vi "Navigation.vi"(0 "output angle":dbl, 4 "output xy":dbl, 6 "Debug":bool, 8 "GoTo Navigation":bool, 11 "IA State Output in":T1) -> (3 "IA State Output out":T1)   [LabVIEW 2018]
uses:
  Core/AI Input.ctl
  Core/AI Robot.ctl
  Intel/Functions Enum.ctl
  Intel/AttackerStates.ctl
  Path Planning/RRT/PathDests.ctl
  Path Planning/RRT/PathDest.ctl
  Core/AI Ball.ctl
  Core/Field Size.ctl
  Core/AI Judge.ctl
  Intel/Command Enum.ctl
  Util/Events/Events.ctl
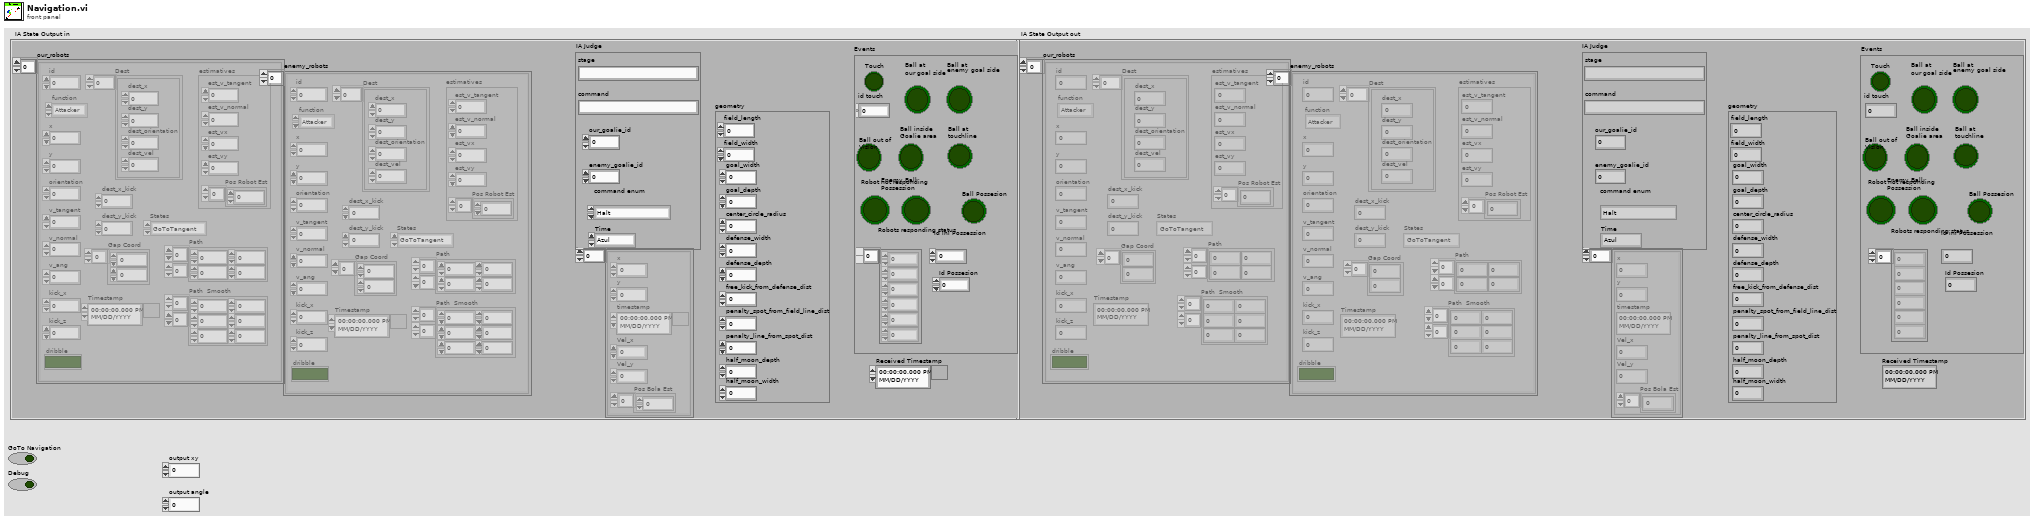
[diagram p1: front panel]
types:
  T1 = typedef "AI Input.ctl" = cluster{"our_robots":T2[], "enemy_robots":T2[], "balls":T7[], "geometry":T8, "IA Judge":T9, "Received Timestamp":timestamp, "Events":T11}
  T2 = typedef "AI Robot.ctl" = cluster{"id":u32, "function":T3, "x":dbl, "y":dbl, "orientation":dbl, "v_tangent":dbl, "v_normal":dbl, "v_ang":dbl, "kick_x":dbl, "kick_z":dbl, "dribble":bool, "Timestamp":timestamp, "estimatives":cluster{"est_v_tangent":dbl, "est_v_normal":dbl, "est_vx":dbl, "est_vy":dbl, "Pos Robot Est":dbl[]}, "dest_x_kick":dbl, "dest_y_kick":dbl, "Gap Coord":dbl[], "States":T4, "Path ":dbl[][], "Path  Smooth":dbl[][], "Dest":T5}
  T3 = typedef "Functions Enum.ctl" = enum16{"Attacker", "Goalie", "Defender", "Striker", "Goto 0", "Dummy", "Kicker", "ZigZag"}
  T4 = typedef "AttackerStates.ctl" = enum16{"Pass", "GoToTangent", "BallGetting", "GoToKick", "Rotate anti-clockwise", "Rotate Clockwise", ""}
  T5 = typedef "PathDests.ctl" = T6[]
  T6 = typedef "PathDest.ctl" = cluster{"dest_x":dbl, "dest_y":dbl, "dest_orientation":dbl, "dest_vel":dbl}
  T7 = typedef "AI Ball.ctl" = cluster{"x":dbl, "y":dbl, "timestamp":timestamp, "Vel_x":dbl, "Vel_y":dbl, "Pos Bola Est":dbl[]}
  T8 = typedef "Field Size.ctl" = cluster{"field_length":u32, "field_width":u32, "goal_width":u32, "goal_depth":u32, "center_circle_radius":u32, "defense_width":u32, "defense_depth":u32, "free_kick_from_defense_dist":u32, "penalty_spot_from_field_line_dist":u32, "penalty_line_from_spot_dist":u32, "half_moon_depth":u32, "half_moon_width":u32}
  T9 = typedef "AI Judge.ctl" = cluster{"stage":string, "command":string, "our_goalie_id":dbl, "enemy_goalie_id":dbl, "command enum":T10, "Time":enum16{"Azul", "Amarelo"}}
  T10 = typedef "Command Enum.ctl" = enum16{"Halt", "Stop", "Force Start", "PKA Normal Start", "Prepare Kickoff Ally", "PKE Normal Start", "Prepare Kickoff Enemy", "Prepare Penalty Ally", "PPA Normal Start", "Prepare Penalty Enemy", "PPE Normal Start", "Ball Placement Enemy Up", "Ball Placement Enemy Down", "Ball Placement Ally Up", "Ball Placement Ally Mid", "Ball Placement Ally Down", "Indirect Free Enemy", "Indirect Free Ally", "Timeout Enemy", "Timeout Ally", "Goal Enemy", "Goal Ally", "Normal Half Time", "Extra Time Break", "Extra Half Time", "None", "Post Game"}
  T11 = typedef "Events.ctl" = cluster{"Touch":bool, "id touch":dbl, "Ball out of \nVision":bool, "Ball inside \nGoalie area":bool, "Robot not responding":bool, "Robots responding status":dbl[], "Enemy Ball \nPossession":bool, "Id ini Possession":dbl, "Ball Possesion":bool, "Id Possesion":dbl, "Ball at\nour goal side":bool, "Ball at\ntouchline":bool, "Ball at\nenemy goal side":bool}
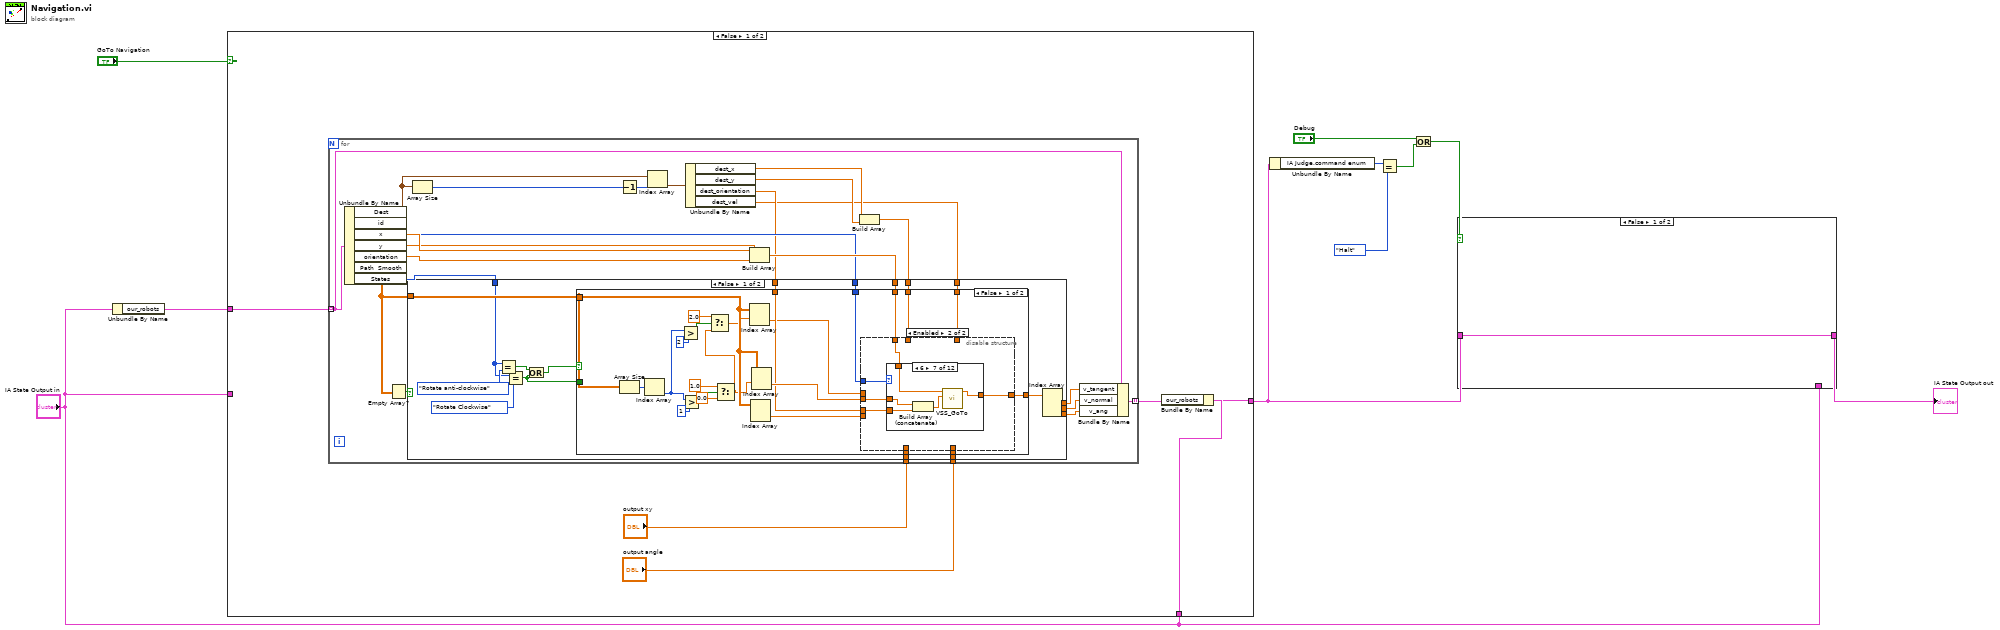
[diagram p0: block diagram]
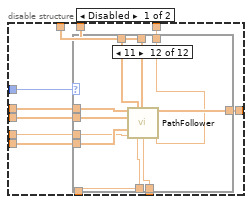
[diagram p2: hidden frame]
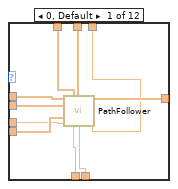
[diagram p3: hidden frame]
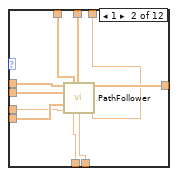
[diagram p4: hidden frame]
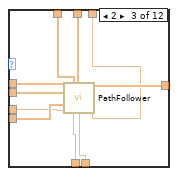
[diagram p5: hidden frame]
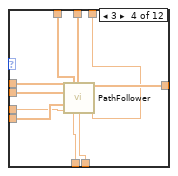
[diagram p6: hidden frame]
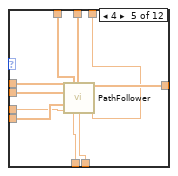
[diagram p7: hidden frame]
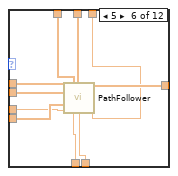
[diagram p8: hidden frame]
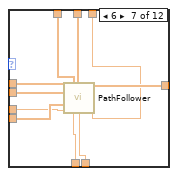
[diagram p9: hidden frame]
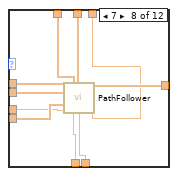
[diagram p10: hidden frame]
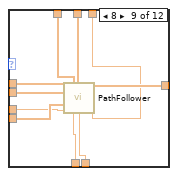
[diagram p11: hidden frame]
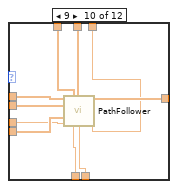
[diagram p12: hidden frame]
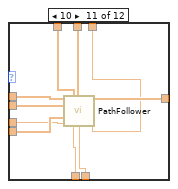
[diagram p13: hidden frame]
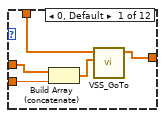
[diagram p14: hidden frame]
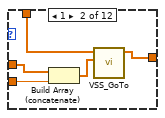
[diagram p15: hidden frame]
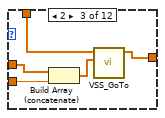
[diagram p16: hidden frame]
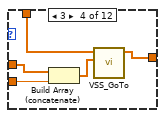
[diagram p17: hidden frame]
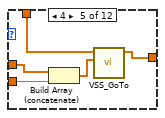
[diagram p18: hidden frame]
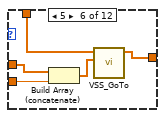
[diagram p19: hidden frame]
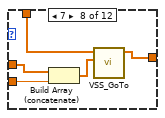
[diagram p20: hidden frame]
diagram:
  n1 = Unbundle By Name("IA State Output in") -> ("our_robots"=w10:T2[])
  n2 = case shown="False" "GoTo Navigation" {
    tunnel: w10 -> [w16 _]
    tunnel: [w13 w285] -> w6
    tunnel: "IA State Output in" -> [_ w286]
    tunnel: "IA State Output in" -> [w14 _]
    frame False {
      n3 = for {
        tunnel: w16 -> [w18] mode=indexing
        tunnel: [w33] -> w15 mode=indexing
        tunnel: "output xy" -> [w31]
        tunnel: "output angle" -> [w30]
        n4 = Unbundle By Name(w18) -> ("Dest"=w28:T5, "id"=w32:u32, "x"=w40:dbl, "y"=w39:dbl, "orientation"=w38:dbl, "Path  Smooth"=w19:dbl[][], "States"=w17:T4)
        n5 = Empty Array?(array=w19) -> (empty?=w20:bool)
        n6 = Array Size(array=w28) -> (size(s)=w27:i32)
        n7 = Decrement(x=w27) -> (x-1=w26:i32)
        n8 = Index Array(array=w28, index=w26) -> (element=w25:T6)
        n9 = Unbundle By Name(w25) -> ("dest_x"=w24:dbl, "dest_y"=w23:dbl, "dest_orientation"=w22:dbl, "dest_vel"=w21:dbl)
        n10 = Build Array(w40, w39, w38) -> (w37:dbl[])
        n11 = Build Array(w24, w23) -> (w29:dbl[])
        n12 = case shown="False" w20 {
          tunnel: w37 -> [w58 _]
          tunnel: [w56 w284] -> w36
          tunnel: [w55 w284] -> w35
          tunnel: [w54 w284] -> w34
          tunnel: w32 -> [w53 _]
          tunnel: w31 -> [w52 _]
          tunnel: w30 -> [w51 _]
          tunnel: w19 -> [w47 _]
          tunnel: w29 -> [w50 _]
          tunnel: w22 -> [w49 _]
          tunnel: w21 -> [w48 _]
          tunnel: w17 -> [w44 _]
          frame False {
            n13 = Equal?(x=w44, y=AttackerStates."Rotate anti-clockwise" ("States")) -> (x = y?=w43:bool)
            n14 = Equal?(x=w44, y=AttackerStates."Rotate Clockwise" ("States")) -> (x = y?=w41:bool)
            n15 = Or(x=w43, y=w41) -> (x .or. y?=w42:bool)
            n16 = case shown="False" w42 {
              tunnel: w58 -> [w81 _]
              tunnel: [w80 w283] -> w57
              tunnel: w53 -> [w74 _]
              tunnel: w52 -> [w71 _]
              tunnel: w51 -> [w70 _]
              tunnel: w50 -> [w69 _]
              tunnel: w49 -> [w68 _]
              tunnel: w48 -> [w67 _]
              tunnel: w47 -> [w63 _]
              tunnel: w41 -> [_ w281]
              frame False {
                n17 = Array Size(array=w63) -> (size(s)=w79:i32[])
                n18 = Index Array(array=w79) -> (element=w60:i32)  [unwired: 1 in]
                n19 = Greater?(x=w60, y=2) -> (0:w64:bool)
                n20 = Greater?(x=w60, y=1) -> (0:w78:bool)
                n21 = Select(t=1.0, s=w78, f=0.0) -> (s? t:f=w61:dbl)
                n22 = Select(t=2.0, s=w64, f=w61) -> (s? t:f=w62:dbl)
                n23 = Index Array(array=w63, index (row)=w62) -> (element=w59:dbl[])  [unwired: 1 in]
                n24 = Index Array(array=w63) -> (element=w72:dbl[])  [unwired: 2 in]
                n25 = Index Array(array=w63, index (row)=w61) -> (element=w73:dbl[])  [unwired: 1 in]
                n26 = disable-structure shown="Enabled" {
                  disable-tunnel: w81 -> [w92 w215]
                  disable-tunnel: [w91 w214] -> w80
                  disable-tunnel: w74 -> [w90 w217]
                  disable-tunnel: w73 -> [w89 w216]
                  disable-tunnel: w72 -> [w88 _]
                  disable-tunnel: w71 -> [w87 _]
                  disable-tunnel: w70 -> [w86 _]
                  disable-tunnel: w69 -> [w85 _]
                  disable-tunnel: w68 -> [w84 w213]
                  disable-tunnel: w67 -> [w83 _]
                  disable-tunnel: w59 -> [w82 _]
                  frame Disabled {
                    n27 = case shown="11" w90 {
                      tunnel: w89 -> [w101 w111 w121 w131 w141 w151 w161 w171 w181 w191 w201 w211]
                      tunnel: w92 -> [w97 w107 w117 w127 w137 w147 w157 w167 w177 w187 w197 w207]
                      tunnel: [w102 w112 w122 w132 w142 w152 w162 w172 w182 w192 w202 w212] -> w91
                      tunnel: w88 -> [w100 w110 w120 w130 w140 w150 w160 w170 w180 w190 w200 w210]
                      tunnel: w87 -> [w99 w109 w119 w129 w139 w149 w159 w169 w179 w189 w199 w209]
                      tunnel: w86 -> [w98 w108 w118 w128 w138 w148 w158 w168 w178 w188 w198 w208]
                      tunnel: w85 -> [w96 w106 w116 w126 w136 w146 w156 w166 w176 w186 w196 w206]
                      tunnel: w84 -> [w95 w105 w115 w125 w135 w145 w155 w165 w175 w185 w195 w205]
                      tunnel: w83 -> [w94 w104 w114 w124 w134 w144 w154 w164 w174 w184 w194 w204]
                      tunnel: w82 -> [w93 w103 w113 w123 w133 w143 w153 w163 w173 w183 w193 w203]
                      frame 0, Default {
                        n28 = call "PathFollower.vi"("Waypoint 2"=w93, "Position"=w97, "Dest"=w96, "Waypoint 1"=w101, "Waypoint 0"=w100, "Dest_orientation"=w95, "output xy"=w99, "output angle"=w98, "dest_vel"=w94) -> ("Output\nVelocity"=w102:dbl[])  [unwired: 6 in]
                      }
                      frame 1 {
                        n29 = call "PathFollower.vi"("Waypoint 2"=w103, "Position"=w107, "Dest"=w106, "Waypoint 1"=w111, "Waypoint 0"=w110, "Dest_orientation"=w105, "output xy"=w109, "output angle"=w108, "dest_vel"=w104) -> ("Output\nVelocity"=w112:dbl[])  [unwired: 6 in]
                      }
                      frame 2 {
                        n30 = call "PathFollower.vi"("Waypoint 2"=w113, "Position"=w117, "Dest"=w116, "Waypoint 1"=w121, "Waypoint 0"=w120, "Dest_orientation"=w115, "output xy"=w119, "output angle"=w118, "dest_vel"=w114) -> ("Output\nVelocity"=w122:dbl[])  [unwired: 6 in]
                      }
                      frame 3 {
                        n31 = call "PathFollower.vi"("Waypoint 2"=w123, "Position"=w127, "Dest"=w126, "Waypoint 1"=w131, "Waypoint 0"=w130, "Dest_orientation"=w125, "output xy"=w129, "output angle"=w128, "dest_vel"=w124) -> ("Output\nVelocity"=w132:dbl[])  [unwired: 6 in]
                      }
                      frame 4 {
                        n32 = call "PathFollower.vi"("Waypoint 2"=w133, "Position"=w137, "Dest"=w136, "Waypoint 1"=w141, "Waypoint 0"=w140, "Dest_orientation"=w135, "output xy"=w139, "output angle"=w138, "dest_vel"=w134) -> ("Output\nVelocity"=w142:dbl[])  [unwired: 6 in]
                      }
                      frame 5 {
                        n33 = call "PathFollower.vi"("Waypoint 2"=w143, "Position"=w147, "Dest"=w146, "Waypoint 1"=w151, "Waypoint 0"=w150, "Dest_orientation"=w145, "output xy"=w149, "output angle"=w148, "dest_vel"=w144) -> ("Output\nVelocity"=w152:dbl[])  [unwired: 6 in]
                      }
                      frame 6 {
                        n34 = call "PathFollower.vi"("Waypoint 2"=w153, "Position"=w157, "Dest"=w156, "Waypoint 1"=w161, "Waypoint 0"=w160, "Dest_orientation"=w155, "output xy"=w159, "output angle"=w158, "dest_vel"=w154) -> ("Output\nVelocity"=w162:dbl[])  [unwired: 6 in]
                      }
                      frame 7 {
                        n35 = call "PathFollower.vi"("Waypoint 2"=w163, "Position"=w167, "Dest"=w166, "Waypoint 1"=w171, "Waypoint 0"=w170, "Dest_orientation"=w165, "output xy"=w169, "output angle"=w168, "dest_vel"=w164) -> ("Output\nVelocity"=w172:dbl[])  [unwired: 6 in]
                      }
                      frame 8 {
                        n36 = call "PathFollower.vi"("Waypoint 2"=w173, "Position"=w177, "Dest"=w176, "Waypoint 1"=w181, "Waypoint 0"=w180, "Dest_orientation"=w175, "output xy"=w179, "output angle"=w178, "dest_vel"=w174) -> ("Output\nVelocity"=w182:dbl[])  [unwired: 6 in]
                      }
                      frame 9 {
                        n37 = call "PathFollower.vi"("Waypoint 2"=w183, "Position"=w187, "Dest"=w186, "Waypoint 1"=w191, "Waypoint 0"=w190, "Dest_orientation"=w185, "output xy"=w189, "output angle"=w188, "dest_vel"=w184) -> ("Output\nVelocity"=w192:dbl[])  [unwired: 6 in]
                      }
                      frame 10 {
                        n38 = call "PathFollower.vi"("Waypoint 2"=w193, "Position"=w197, "Dest"=w196, "Waypoint 1"=w201, "Waypoint 0"=w200, "Dest_orientation"=w195, "output xy"=w199, "output angle"=w198, "dest_vel"=w194) -> ("Output\nVelocity"=w202:dbl[])  [unwired: 6 in]
                      }
                      frame 11 {
                        n39 = call "PathFollower.vi"("Waypoint 2"=w203, "Position"=w207, "Dest"=w206, "Waypoint 1"=w211, "Waypoint 0"=w210, "Dest_orientation"=w205, "output xy"=w209, "output angle"=w208, "dest_vel"=w204) -> ("Output\nVelocity"=w212:dbl[])  [unwired: 6 in]
                      }
                    }
                  }
                  frame Enabled {
                    n40 = case shown="6" w217 {
                      tunnel: w216 -> [w220 w225 w230 w235 w240 w245 w250 w255 w260 w265 w270 w275]
                      tunnel: w215 -> [w222 w227 w232 w237 w242 w247 w252 w257 w262 w267 w272 w277]
                      tunnel: [w221 w226 w231 w236 w241 w246 w251 w256 w261 w266 w271 w276] -> w214
                      tunnel: w213 -> [w219 w224 w229 w234 w239 w244 w249 w254 w259 w264 w269 w274]
                      frame 0, Default {
                        n41 = Build Array (concatenate)(w220, w219) -> (w218:dbl[])
                        n42 = call "VSS_GoTo.vi"("SetPoint"=w218, "Position"=w222) -> ("Output Vel"=w221:dbl[])  [unwired: 9 in]
                      }
                      frame 1 {
                        n43 = Build Array (concatenate)(w225, w224) -> (w223:dbl[])
                        n44 = call "VSS_GoTo.vi"("SetPoint"=w223, "Position"=w227) -> ("Output Vel"=w226:dbl[])  [unwired: 9 in]
                      }
                      frame 2 {
                        n45 = Build Array (concatenate)(w230, w229) -> (w228:dbl[])
                        n46 = call "VSS_GoTo.vi"("SetPoint"=w228, "Position"=w232) -> ("Output Vel"=w231:dbl[])  [unwired: 9 in]
                      }
                      frame 3 {
                        n47 = Build Array (concatenate)(w235, w234) -> (w233:dbl[])
                        n48 = call "VSS_GoTo.vi"("SetPoint"=w233, "Position"=w237) -> ("Output Vel"=w236:dbl[])  [unwired: 9 in]
                      }
                      frame 4 {
                        n49 = Build Array (concatenate)(w240, w239) -> (w238:dbl[])
                        n50 = call "VSS_GoTo.vi"("SetPoint"=w238, "Position"=w242) -> ("Output Vel"=w241:dbl[])  [unwired: 9 in]
                      }
                      frame 5 {
                        n51 = Build Array (concatenate)(w245, w244) -> (w243:dbl[])
                        n52 = call "VSS_GoTo.vi"("SetPoint"=w243, "Position"=w247) -> ("Output Vel"=w246:dbl[])  [unwired: 9 in]
                      }
                      frame 6 {
                        n53 = Build Array (concatenate)(w250, w249) -> (w248:dbl[])
                        n54 = call "VSS_GoTo.vi"("SetPoint"=w248, "Position"=w252) -> ("Output Vel"=w251:dbl[])  [unwired: 9 in]
                      }
                      frame 7 {
                        n55 = Build Array (concatenate)(w255, w254) -> (w253:dbl[])
                        n56 = call "VSS_GoTo.vi"("SetPoint"=w253, "Position"=w257) -> ("Output Vel"=w256:dbl[])  [unwired: 9 in]
                      }
                      frame 8 {
                        n57 = Build Array (concatenate)(w260, w259) -> (w258:dbl[])
                        n58 = call "VSS_GoTo.vi"("SetPoint"=w258, "Position"=w262) -> ("Output Vel"=w261:dbl[])  [unwired: 9 in]
                      }
                      frame 9 {
                        n59 = Build Array (concatenate)(w265, w264) -> (w263:dbl[])
                        n60 = call "VSS_GoTo.vi"("SetPoint"=w263, "Position"=w267) -> ("Output Vel"=w266:dbl[])  [unwired: 9 in]
                      }
                      frame 10 {
                        n61 = Build Array (concatenate)(w270, w269) -> (w268:dbl[])
                        n62 = call "VSS_GoTo.vi"("SetPoint"=w268, "Position"=w272) -> ("Output Vel"=w271:dbl[])  [unwired: 9 in]
                      }
                      frame 11 {
                        n63 = Build Array (concatenate)(w275, w274) -> (w273:dbl[])
                        n64 = call "VSS_GoTo.vi"("SetPoint"=w273, "Position"=w277) -> ("Output Vel"=w276:dbl[])  [unwired: 9 in]
                      }
                    }
                  }
                }
              }
              frame True {
                w279 = 3.0 ("element")
                w282 = 0.0 ("element")
                n65 = Negate(x=w279) -> (-x=w280:dbl)
                n66 = Select(t=w279, s=w281, f=w280) -> (s? t:f=w278:dbl)
                n67 = Build Array(w282, w282, w278) -> (w283:dbl[])
              }
            }
            n68 = Index Array(array=w57) -> (element #1=w56:dbl, element #2=w55:dbl, element #3=w54:dbl)  [unwired: 3 in]
          }
          frame True {
            w284 = 0.0 ("output")
          }
        }
        n69 = Bundle By Name(cluster=w18, "v_tangent"=w36, "v_normal"=w35, "v_ang"=w34) -> (w33:T2)
      }
      n70 = Bundle By Name(cluster=w14, "our_robots"=w15) -> (w13:T1)
    }
    frame True {
      n71 = call "potential-field.vi"("IA State Output in"=w286) -> ("IA State Output out"=w285:T1)  [unwired: 10 in]
    }
  }
  n72 = Unbundle By Name(w6) -> ("IA Judge.command enum"=w5:T10)
  n73 = Equal?(x=w5, y=Command_Enum."Halt") -> (x = y?=w2:bool)
  n74 = Or(x="Debug", y=w2) -> (x .or. y?=w3:bool)
  n75 = case shown="False" w3 {
    tunnel: [w287 w292] -> w8
    tunnel: w6 -> [w287 w289]
    tunnel: "IA State Output in" -> [_ w290]
    frame False {
    }
    frame True {
      n76 = Unbundle By Name(w289) -> ("our_robots"=w288:T2[])
      n77 = for {
        tunnel: [w295] -> w291 mode=indexing
        tunnel: w288 -> [w293] mode=indexing
        w294 = 0.0 ("v_normal")
        n78 = Bundle By Name(cluster=w293, "v_tangent"=w294, "v_normal"=w294, "v_ang"=w294) -> (w295:T2)
      }
      n79 = Bundle By Name(cluster=w290, "our_robots"=w291) -> (w292:T1)
    }
  }
  "IA State Output out" <- w8
